vi "Write atime and mtime.vi"(8 "error in (no error)":errorcluster, 10 "atime/mtime":cluster{"atime":u32, "mtime":u32}, 11 "file attributes in":refnum<class "File Attributes.lvclass">) -> (0 "error out":errorcluster, 3 "file attributes out":refnum<class "File Attributes.lvclass">)   [LabVIEW 2020, in "NI_SFTP.lvlib" / "File Attributes.lvclass"]
doc: "Updates the access and modification time stored in this File Attributes object using Unix timestamps. Due to limitations in the SFTP API, the access and modification time must be updated together."
uses:
  <vilib>/net/SFTP/File Attributes/File Attributes.lvclass
  <vilib>/net/SFTP/File Attributes/File Attributes.lvclass/File Attributes.ctl
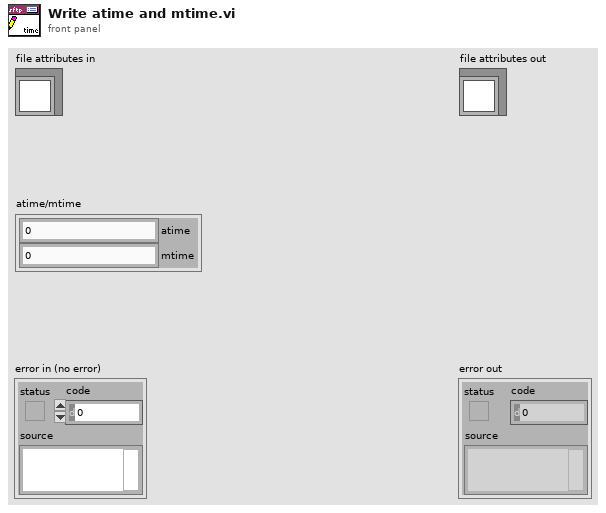
[diagram p1: front panel]
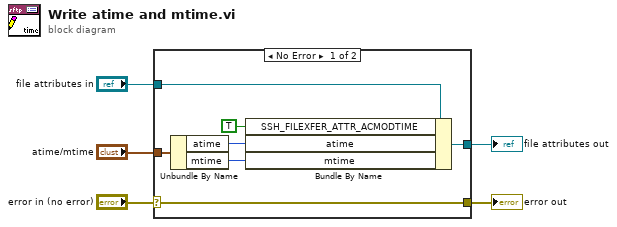
[diagram p0: block diagram]
diagram:
  n1 = case shown="No Error" "error in (no error)" {
    selector: "error in (no error)" -> [w12 w13]
    tunnel: [w12 w13] -> w4
    tunnel: [w10 w14] -> w2
    tunnel: "file attributes in" -> [w11 w14]
    tunnel: "atime/mtime" -> [w9 _]
    frame No Error {
      n2 = Unbundle By Name(w9) -> ("atime"=w8:u32, "mtime"=w7:u32)
      n3 = Bundle By Name(cluster=w11, "SSH_FILEXFER_ATTR_ACMODTIME"=TRUE ("SFTP Session.lvclass:Name.File Attributes.SSH_FILEXFER_ATTR_ACMODTIME"), "atime"=w8, "mtime"=w7) -> (w10:refnum<class "File Attributes.lvclass">)
    }
    frame Error {
    }
  }
  "error out" <- w4
  "file attributes out" <- w2
